vi "GOOP_LVClass_Provider_Interface.vi"() -> (3 "Interface Table":T1)   [LabVIEW 2016]
uses:
  <resource>/Framework/Providers/API/Provider_Interface.ctl
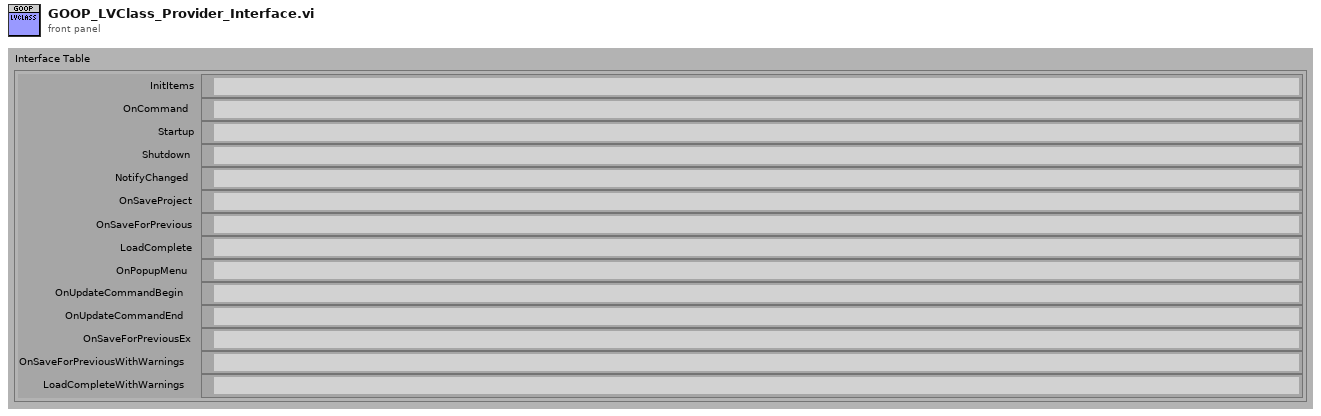
[diagram p1: front panel]
types:
  T1 = typedef "Provider_Interface.ctl" = cluster{"InitItems":path, "OnCommand":path, "Startup":path, "Shutdown":path, "NotifyChanged":path, "OnSaveProject":path, "OnSaveForPrevious":path, "LoadComplete":path, "OnPopupMenu":path, "OnUpdateCommandBegin":path, "OnUpdateCommandEnd":path, "OnSaveForPreviousEx":path, "OnSaveForPreviousWithWarnings":path, "LoadCompleteWithWarnings":path}
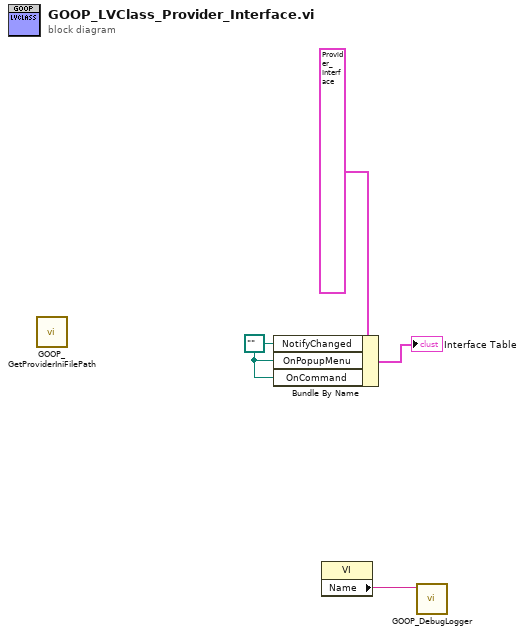
[diagram p0: block diagram]
diagram:
  w1 = path "" ("NotifyChanged")
  n1 = call <resource>:"GOOP_GetProviderIniFilePath.vi"() -> ()  [unwired: 10 in, 2 out]
  n2 = Bundle By Name(cluster=T1 {"InitItems"=path "", "OnCommand"=path "", "Startup"=path "", "Shutdown"=path "", "NotifyChanged"=path "", "OnSaveProject"=path "", "OnSaveForPrevious"=path "", "LoadComplete"=path "", "OnPopupMenu"=path "", "OnUpdateCommandBegin"=path "", "OnUpdateCommandEnd"=path "", "OnSaveForPreviousEx"=path "", "OnSaveForPreviousWithWarnings"=path "", "LoadCompleteWithWarnings"=path ""} ("InterfaceTable"), "NotifyChanged"=w1, "OnPopupMenu"=w1, "OnCommand"=w1) -> (→"Interface Table":T1)
  n3 = property class="VI"() -> ("Name"=w2:string)  [unwired: 2 in, 2 out]
  n4 = call <resource>:"GOOP_DebugLogger.vi"("State"=w2) -> ()  [unwired: 8 in, 3 out]
